vi "Convert Hex to ASCII.vi"(1 "Offset (0)":u32, 2 "Hex String":string) -> (0 "ASCII String":string)   [LabVIEW 2024, in "Bronkhorst FLOW-BUS.lvlib"]
doc: "Converts the input HEX String to an ASCII String and outputs it. This is used to decode ASCII Strings from the instruments response."
uses:
  Bronkhorst FLOW-BUS.lvlib
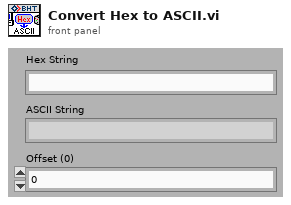
[diagram p1: front panel]
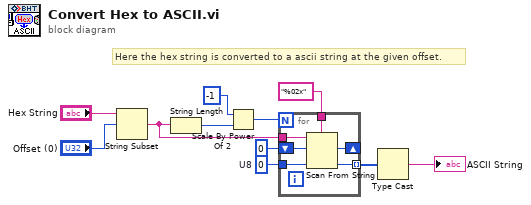
[diagram p0: block diagram]
diagram:
  w11 = u8 0  # U8
  # "Here the hex string is converted to a ascii string at the given offset."
  n1 = String Subset(string="Hex String", offset (0)="Offset (0)") -> (substring=w2:string)  [unwired: 1 in]
  n2 = String Length(string=w2) -> (length=w6:i32)
  n3 = Scale By Power Of 2(n=-1, x=w6) -> (x*2^n=w7:i32)
  n4 = for {
    N: w7 -> [_]
    shift-right: [w16] -> _
    shift-left: u32 0 -> [w17]
    tunnel: w11 -> [w15]
    tunnel: "%02x" ("format string") -> [w14]
    tunnel: [w13] -> w5 mode=indexing
    tunnel: w2 -> [w12]
    n5 = Scan From String(format string=w14, input string=w12, initial scan location=w17, default 1=w15) -> (offset past scan=w16:u32, output 1=w13:u8)  [unwired: 1 in, 2 out]
  }
  n6 = Type Cast(x=w5) -> (*(type *) &x=→"ASCII String":string)  [unwired: 1 in]
